vi "Write additional files.vi"(8 "error in":errorcluster, 10 "additional files":T1[](array[typedef]), 11 "Targets in":refnum<class "Targets.lvclass">) -> (0 "error out":errorcluster, 3 "Targets out":refnum<class "Targets.lvclass">)   [LabVIEW 2013, in "PL Framework Configuration Tool.lvlib" / "Targets.lvclass"]
uses:
  Targets.lvclass
  TBM Configuration Node/deployment configuration.ctl
  Targets.lvclass/Targets.ctl
  TBM Configuration Node/TBM Configuration Node.lvclass
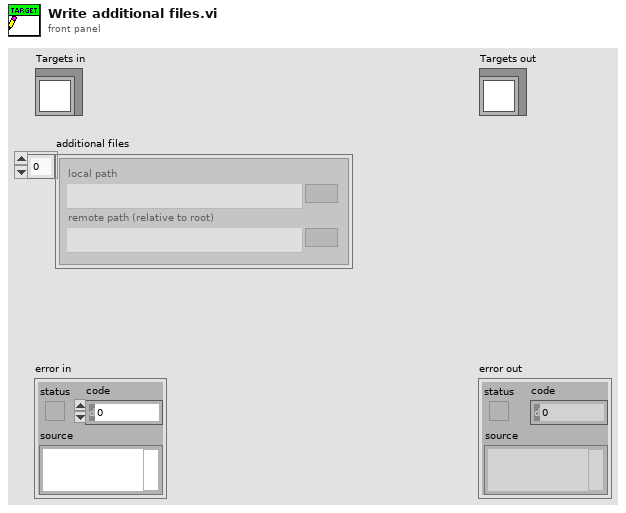
[diagram p1: front panel]
types:
  T1 = typedef "PL Framework Configuration Tool.lvlib/TBM Configuration Node.lvclass/deployment configuration.ctl" = cluster{"local path":path, "remote path (relative to root)":path}
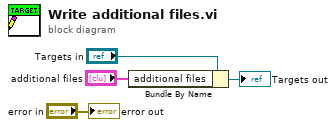
[diagram p0: block diagram]
diagram:
  n1 = Bundle By Name(cluster="Targets in", "additional files"="additional files") -> (→"Targets out":refnum<class "Targets.lvclass">)
  "error out" <- "error in"
